vi "Comparation.vi"() -> ()   [LabVIEW 2018]
uses:
  MainFGV/Settings/Advanced/AdvancedConfig.ctl
  Processing/GraphMean/plot_props.ctl
  Processing/GraphMean/axis_props.ctl
  <vilib>/Heliosphere Research LLC/Advanced Plotting Toolkit/api_core/NewPlotScales.ctl
  Processing/results_data.ctl
  Processing/GraphMean/data_mean_plot.ctl
  <vilib>/Analysis/NI_AALPro.lvlib
  <vilib>/Heliosphere Research LLC/Advanced Plotting Toolkit/Advanced Plotting Toolkit.lvlib
panel:
  in  "order":i32=2 caption="Ordem suavização" min=2 max=20
  in  "freq_suav":dbl(slide) caption="Frequência suavização" scale=0.1..0.5
  in  "peakMode":bool
  in  "ranges":T1(array[cluster])=[{"minFreq"=0.0, "maxFreq"=1000.0, "alpha"=20.0}] caption="Ranges de procura de picos" {"alpha" min=0.0 max=100.0 format="%#_6f %"; "maxFreq" format="%#_g Hz"; "minFreq" format="%#_g Hz"}
  in  "Ensaios":path=path "C:/Users/l01481/Desktop/nada"
  in  "channel":i32=1 caption="Canal" min=1 max=4
  in  "stop":bool
  in  "log":bool
  in  "alpha":dbl=0.3 caption="Alpha" format="%#_6f"
  in  "maxFreq":dbl=72.0 caption="Frequência máxima" format="%#_g Hz"
  in  "minFreq":dbl=30.0 caption="Frequência mínima" format="%#_g Hz"
  in  "lowPass":dbl=1000.0 caption="Passa baixa" format="%#_g Hz"
  in  "highPass":dbl=1.0 caption="Passa alta" format="%#_g Hz"
  in  "Filtro":T2(ring)=enum."Passa banda"
  in  "cutoff":dbl=-6.0 caption="Cutoff amplitude [dB]" format="%#_g dB"
  in  "delete":bool
  in  "ok":bool
  in  "validate":bool
  in  "tab":T3(tab)
  out "inert":waveform(dbl)[](graph) caption="Inertância"
  out "hammerSpec":waveform(dbl)(graph) caption="Martelo - Espectro"
  out "acelTime":waveform(dbl)[](graph) caption="Acelerômetros - Sinal no tempo"
  out "hammerTime":waveform(dbl)(graph) caption="Martelo - Sinal no tempo"
  out "meanInert":picture
  out "Picos":cluster{"freqs":dbl[], "Array":dbl[]}[](graph) caption="XY Graph"
  out "Frequências":dbl[][](array[numeric])
  out "Picos 2":cluster{"freqs":dbl[], "Array":dbl[]}[](graph) caption="XY Graph"
  # "Análise modal\n\nAquisição\n\nLink do repositório: https://github.com/LeonardoSirino/ModalAnalysis"
  # "Leonardo Sirino\nSistemas Mecânicos \nT + 55 (41) 3361-6152 | C + 55 (41) 99679-007\nleonardo.sirino@lactec.org.br | www.lactec.org.br"
  # "Configurações para\napresentação"
  # "Configurações para\nprocessamento"
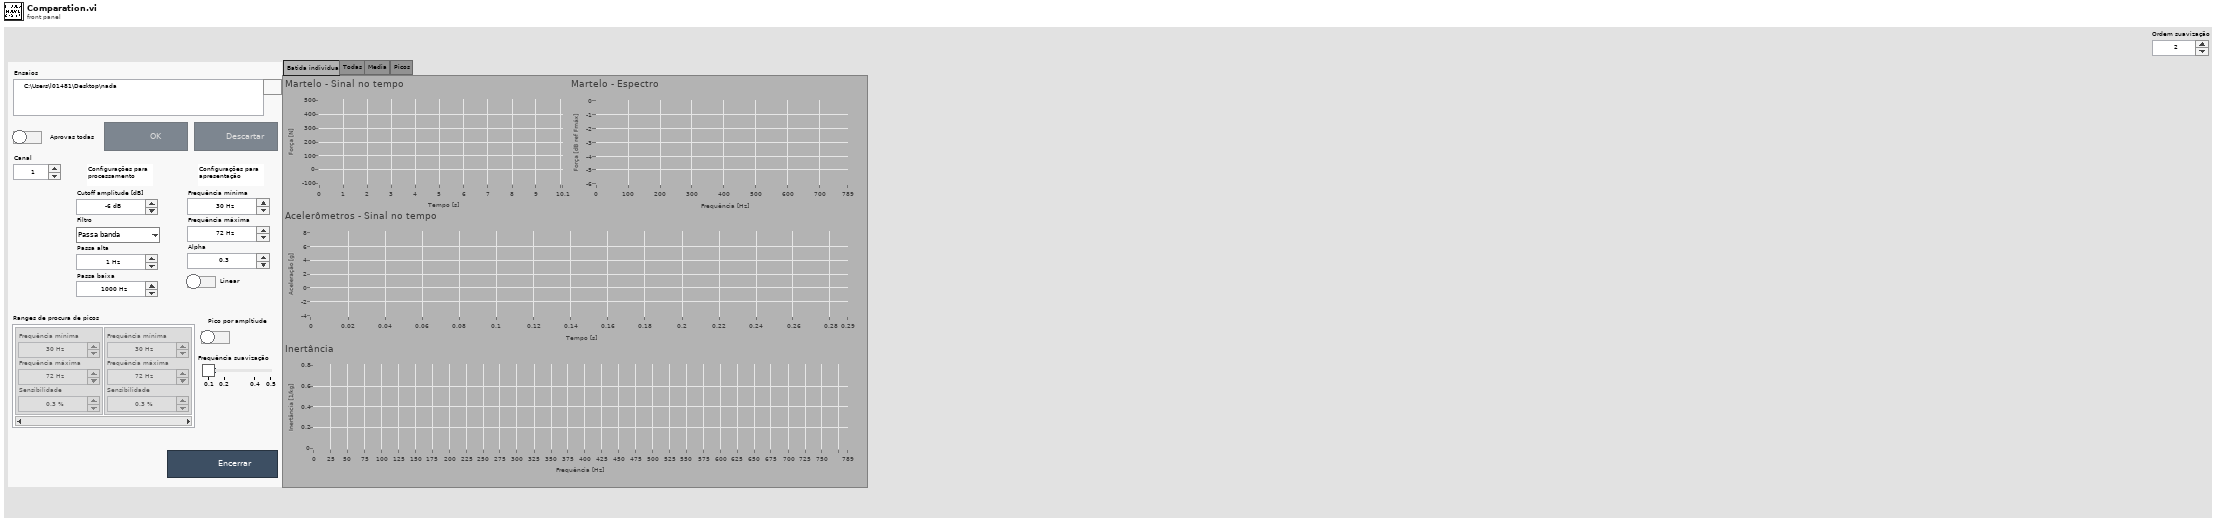
[diagram p1: front panel]
types:
  T1 = cluster{"minFreq":dbl, "maxFreq":dbl, "alpha":dbl}[]
  T2 = enum16{"Desativado", "Passa banda", "Passa alta", "Passa baixa"}
  T3 = enum32{"Batida individual", "Todas", "Media", "Picos"}
  T4 = typedef "plot_props.ctl" = cluster{"x_axis":T5, "y_axis":T5, "y multiplier":dbl, "alpha":dbl, "base_tag":string, "itens_base_name":string, "graph_title":string, "plot_names":string[], "plot_all":bool}
  T5 = typedef "axis_props.ctl" = cluster{"min":dbl, "max":dbl, "label":string, "scale":T6}
  T6 = typedef "Advanced Plotting Toolkit.lvlib/NewPlotScales.ctl" = enum16{"Default", "Linear", "Log", "Symlog"}
  T7 = enum8{"Enabled", "Disabled", "Disabled and Grayed Out"}
  T8 = typedef "AdvancedConfig.ctl" = cluster{"rate":dbl, "duration":dbl, "thr":dbl, "preTrigger":dbl, "cutoff":dbl, "Filtro":enum16{"Desativado", "Passa banda", "Passa alta", "Passa baixa"}, "highPass":dbl, "lowPass":dbl, "updateTime":dbl}
  T9 = typedef "results_data.ctl" = cluster{"config":T8, "hammer":waveform(dbl), "acelerometers":waveform(dbl)[], "hammerIndex":i32}
  T10 = cluster{"seconds since 1Jan1904":timestamp, "data_out":T9}
  T11 = typedef "data_mean_plot.ctl" = cluster{"array":dbl[], "dx":dbl, "x0":dbl}
  T12 = cluster{"seconds since 1Jan1904":timestamp, "data_out":T9}[]
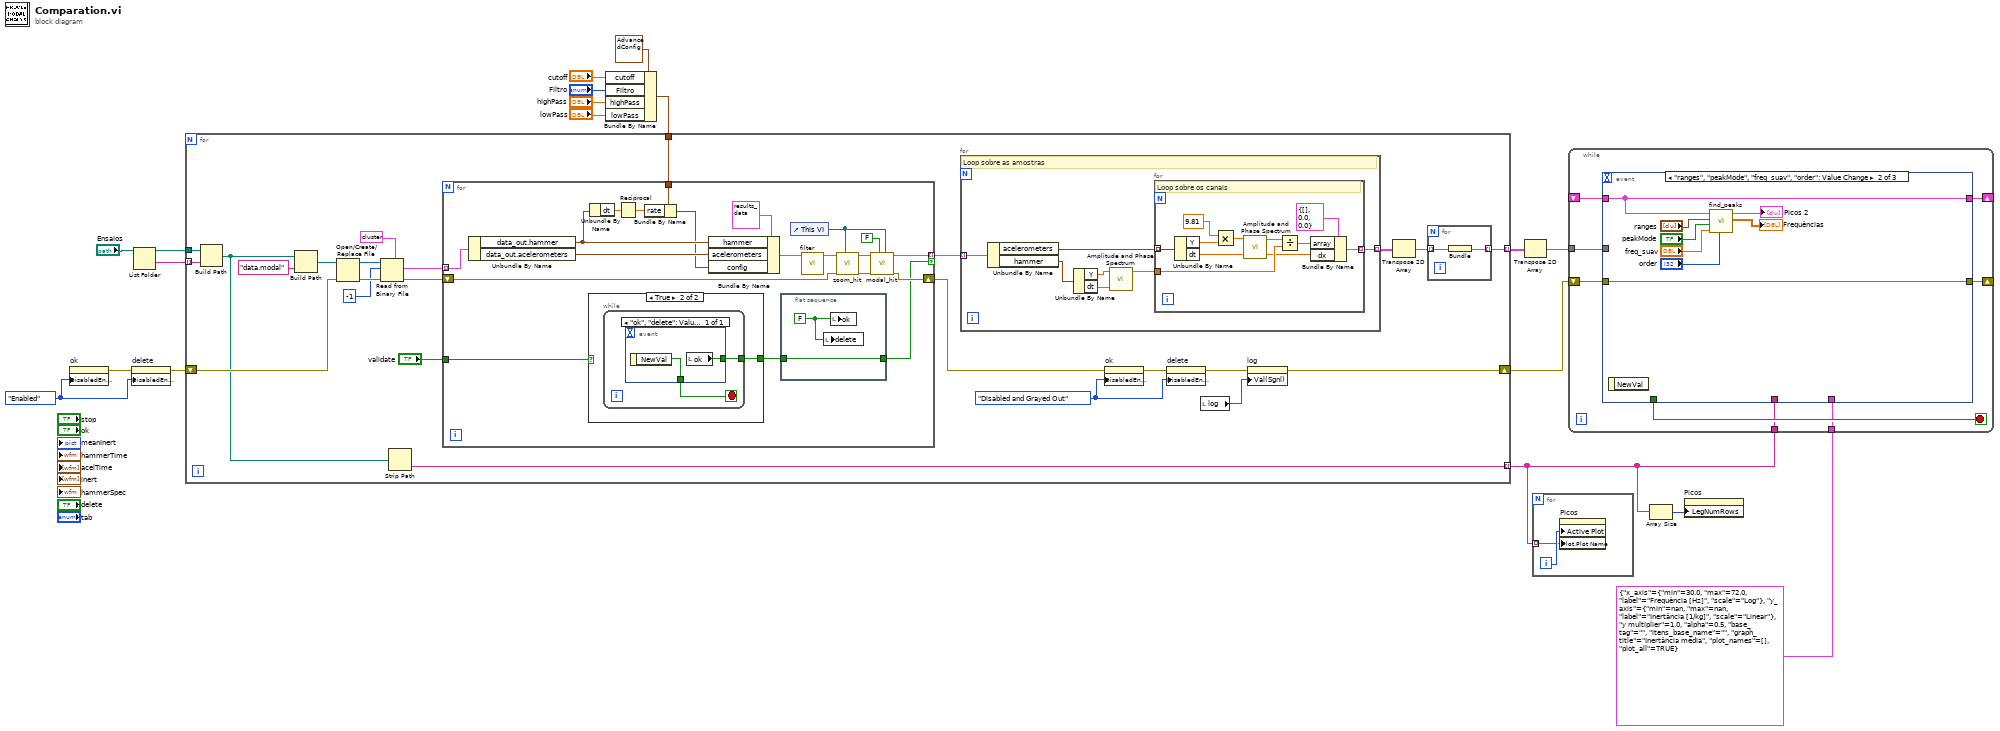
[diagram p0: block diagram]
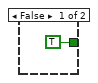
[diagram p2: hidden frame]
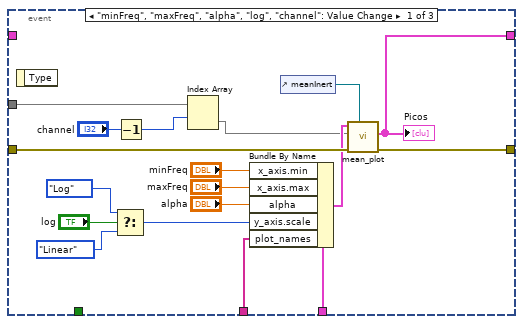
[diagram p3: hidden frame]
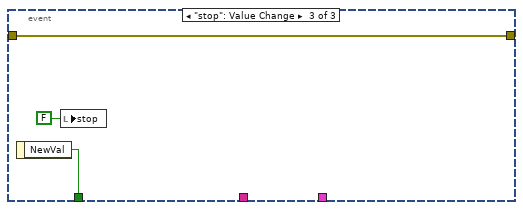
[diagram p4: hidden frame]
diagram:
  w11 = T7."Enabled" ("Disabled")
  n1 = property on="ok" class="Bool (strict)"("DisabledEnum"=w11) -> (error out=w10:errorcluster)  [unwired: 2 in, 1 out]
  n2 = property on="delete" class="Bool (strict)"(error in=w10, "DisabledEnum"=w11) -> (error out=w9:errorcluster)  [unwired: 1 in, 1 out]
  n3 = List Folder(path="Ensaios") -> (path out=w2:path, folder names=w1:string[])  [unwired: 3 in, 2 out]
  n4 = Bundle By Name(cluster=T8 {"rate"=1652.0, "duration"=1.0, "thr"=10.0, "preTrigger"=100.0, "cutoff"=-6.0, "Filtro"=enum."Passa banda", "highPass"=1.0, "lowPass"=1000.0, "updateTime"=50.0} ("config"), "cutoff"="cutoff", "Filtro"="Filtro", "highPass"="highPass", "lowPass"="lowPass") -> (w13:T8)
  n5 = for {
    tunnel: w13 -> [w36]
    tunnel: [w28] -> w8 mode=indexing
    shift-right: [w29] -> w12
    shift-left: w9 -> [w23]
    tunnel: w2 -> [w21]
    tunnel: [w22] -> w6 mode=indexing
    tunnel: w1 -> [w20] mode=indexing
    w25 = T7."Disabled and Grayed Out" ("Disabled")
    n6 = Build Path(base path=w21, name or relative path=w20) -> (appended path=w19:path)
    n7 = Build Path(base path=w19, name or relative path="data.modal") -> (appended path=w42:path)
    n8 = Open/Create/Replace File(file path (use dialog)=w42, error in=w23) -> (refnum out=w41:refnum<file>, error out=w39:errorcluster)  [unwired: 4 in, 1 out]
    n9 = Read from Binary File(5:T10 {"seconds since 1Jan1904"=timestamp(0 s since 1904-01-01), "data_out"={"config"={"rate"=0.0, "duration"=0.0, "thr"=0.0, "preTrigger"=0.0, "cutoff"=0.0, "Filtro"=enum."Desativado", "highPass"=0.0, "lowPass"=0.0, "updateTime"=0.0}, "hammer"={"t0"=timestamp(0 s since 1904-01-01), "dt"=1.0, "Y"=[]}, "acelerometers"=[], "hammerIndex"=0}} ("output cluster"), 8:w39, 10:-1 ("count (1)"), 11:w41) -> (0:w35:errorcluster, 2:w37:T12)  [unwired: 2 in, 2 out]
    n10 = Strip Path(path=w19) -> (name=w22:string)  [unwired: 1 out]
    n11 = for {
      tunnel: w37 -> [w83] mode=indexing
      tunnel: w36 -> [w73]
      shift-right: [w68] -> w27
      shift-left: w35 -> [w69]
      tunnel: [w66] -> w33 mode=indexing if=w65
      tunnel: "validate" -> [w64]
      n12 = Unbundle By Name(w83) -> ("data_out.hammer"=w74:waveform(dbl), "data_out.acelerometers"=w78:waveform(dbl)[])
      n13 = case shown="True" w64 {
        tunnel: [TRUE ("ok") w87] -> w67
        frame False {
        }
        frame True {
          n14 = while {
            tunnel: [w89] -> w87
            stop <- w88 stop-if-true
            n15 = event shown="[0] \"ok\", \"delete\": Value Change" {
              selector: _ -> [_]
              dyn-events: _ -> [_]
              timeout: _ -> [_]
              tunnel: [w90] -> w89
              tunnel: [w91] -> w88
              event "ok", "delete": Value Change {
                n16 = event-data() -> ("NewVal"=w91:bool)  [unwired: 1 in]
                n17 = local read "ok"() -> (w90:bool)
              }
            }
          }
        }
      }
      n18 = Unbundle By Name(w74) -> ("dt"=w72:dbl)
      n19 = Reciprocal(x=w72) -> (1/x=w71:dbl)
      n20 = Bundle By Name(cluster=w73, "rate"=w71) -> (w70:T8)
      n21 = Bundle By Name(cluster=T9 {"config"={"rate"=0.0, "duration"=0.0, "thr"=0.0, "preTrigger"=0.0, "cutoff"=0.0, "Filtro"=enum."Desativado", "highPass"=0.0, "lowPass"=0.0, "updateTime"=0.0}, "hammer"={"t0"=timestamp(0 s since 1904-01-01), "dt"=1.0, "Y"=[]}, "acelerometers"=[], "hammerIndex"=0} ("data_in"), "hammer"=w74, "acelerometers"=w78, "config"=w70) -> (w77:T9)
      n22 = flat-sequence {
        tunnel: w67 -> [w85]
        tunnel: [w85] -> w65
        frame #0 {
          w84 = FALSE ("ok")
          n23 = local write "delete"(w84) -> ()
          n24 = local write "ok"(w84) -> ()
        }
      }
      n25 = control-ref of="This VI"() -> (w76:refnum<vi>)
      n26 = call "filter.vi"("data_in"=w77) -> ("data_out"=w80:T9)  [unwired: 9 in, 1 out]
      n27 = call "zoom_hit.vi"("refVI"=w76, "error in"=w69, "data_in"=w80) -> ("error out"=w81:errorcluster, "data_out"=w82:T9)  [unwired: 7 in]
      n28 = call "modal_hit.vi"("refVI"=w76, "acquisition"=FALSE, "error in"=w81, "data_in"=w82) -> ("error out"=w68:errorcluster, "data_out"=w66:T9)  [unwired: 6 in]
    }
    n29 = for {
      tunnel: w33 -> [w52] mode=indexing
      tunnel: [w46] -> w32 mode=indexing
      # "Loop sobre as amostras"
      n30 = Unbundle By Name(w52) -> ("acelerometers"=w51:waveform(dbl)[], "hammer"=w48:waveform(dbl))
      n31 = Unbundle By Name(w48) -> ("Y"=w49:dbl[], "dt"=w50:dbl)
      n32 = call <vilib>:"Amplitude and Phase Spectrum.vi"("dt"=w50, "Signal (V)"=w49) -> ("Amp Spectrum Mag (Vrms)"=w47:dbl[])  [unwired: 1 in, 2 out]
      n33 = for {
        tunnel: w51 -> [w63] mode=indexing
        tunnel: w47 -> [w57]
        tunnel: [w53] -> w46 mode=indexing
        # "Loop sobre os canais"
        n34 = Unbundle By Name(w63) -> ("Y"=w62:dbl[], "dt"=w59:dbl)
        n35 = Multiply(x=9.81, y=w62) -> (x*y=w60:dbl[])
        n36 = call <vilib>:"Amplitude and Phase Spectrum.vi"("dt"=w59, "Signal (V)"=w60) -> ("df"=w54:dbl, "Amp Spectrum Mag (Vrms)"=w58:dbl[])  [unwired: 1 in, 1 out]
        n37 = Divide(x=w58, y=w57) -> (x/y=w55:dbl[])
        n38 = Bundle By Name(cluster=T11 {"array"=[], "dx"=0.0, "x0"=0.0} ("data_mean_plot"), "array"=w55, "dx"=w54) -> (w53:T11)
      }
    }
    n39 = property on="ok" class="Bool (strict)"(error in=w27, "DisabledEnum"=w25) -> (error out=w26:errorcluster)  [unwired: 1 in, 1 out]
    n40 = property on="delete" class="Bool (strict)"(error in=w26, "DisabledEnum"=w25) -> (error out=w24:errorcluster)  [unwired: 1 in, 1 out]
    n41 = local read "log"() -> (w30:bool)
    n42 = property on="log" class="Bool (strict)"(error in=w24, "Val(Sgnl)"=w30) -> (error out=w29:errorcluster)  [unwired: 1 in, 1 out]
    n43 = Transpose 2D Array(2D array=w32) -> (transposed array=w31:T11[][])
    n44 = for {
      tunnel: w31 -> [w45] mode=indexing
      tunnel: [w44] -> w28 mode=indexing
      n45 = Bundle(w45) -> (w44:cluster{T11[]})  [unwired: 1 in]
    }
  }
  n46 = Transpose 2D Array(2D array=w8) -> (transposed array=w7:cluster{T11[]}[][])
  n47 = for {
    tunnel: w6 -> [w92] mode=indexing
    i -> [w93]
    n48 = property on="Picos" class="XYGraph (strict)"("Active Plot"=w93, "Plot.Plot Name"=w92) -> ()  [unwired: 2 in, 2 out]
  }
  n49 = while {
    shift-right: [w100] -> _
    shift-left: _ -> [w101]
    shift-right: [w99] -> _
    shift-left: w12 -> [w98]
    tunnel: w7 -> [w96]
    tunnel: w6 -> [w95]
    tunnel: T4 {"x_axis"={"min"=30.0, "max"=72.0, "label"="Frequência [Hz]", "scale"=enum."Log"}, "y_axis"={"min"=nan, "max"=nan, "label"="Inertância [1/kg]", "scale"=enum."Linear"}, "y multiplier"=1.0, "alpha"=0.5, "base_tag"="", "itens_base_name"="", "graph_title"="Inertância média", "plot_names"=[], "plot_all"=TRUE} ("plot_properties") -> [w94]
    stop <- w97 stop-if-true
    n50 = event shown="[1] \"ranges\", \"peakMode\", \"freq_suav\", \"order\": Value Change" {
      selector: _ -> [_ _ _]
      dyn-events: _ -> [_ _ _]
      timeout: _ -> [_ _ _]
      tunnel: w101 -> [_ w126 _]
      tunnel: [w105 w126 _] -> w100
      tunnel: [w109 w125 w129] -> w99
      tunnel: w98 -> [w118 w125 w129]
      tunnel: [_ _ w130] -> w97
      tunnel: w96 -> [w108 _ _]
      tunnel: w95 -> [w104 _ _]
      tunnel: w94 -> [w102 _ _]
      event "minFreq", "maxFreq", "alpha", "log", "channel": Value Change {
        n51 = event-data() -> ()  [unwired: 1 in, 1 out]
        n52 = Select(t=NewPlotScales."Log" ("y_axis.scale"), s="log", f=NewPlotScales."Linear" ("y_axis.scale")) -> (s? t:f=w117:T6)
        n53 = Decrement(x="channel") -> (x-1=w103:i32)
        n54 = Index Array(array=w108, index (row)=w103) -> (element=w107:cluster{T11[]}[])  [unwired: 1 in]
        n55 = Bundle By Name(cluster=w102, "x_axis.min"="minFreq", "x_axis.max"="maxFreq", "alpha"="alpha", "y_axis.scale"=w117, "plot_names"=w104) -> (w110:T4)
        n56 = control-ref of="meanInert"() -> (w119:refnum<vi>)
        n57 = call "mean_plot.vi"("ref_picture"=w119, "error in"=w118, "channels"=w107, "plot_properties"=w110) -> ("error out"=w109:errorcluster, "mean_curves"=w105:cluster{"freqs":dbl[], "Array":dbl[]}[])  [unwired: 5 in, 1 out]
        "Picos" <- w105
      }
      event "ranges", "peakMode", "freq_suav", "order": Value Change {
        n58 = event-data() -> ()  [unwired: 1 in, 1 out]
        n59 = call "find_peaks.vi"("order"="order", "freq"="freq_suav", "derivativePeak"="peakMode", "ranges"="ranges", "data"=w126) -> ("freqs"=→"Frequências":dbl[][], "plots"=→"Picos 2":cluster{"Array":dbl[], "Array":dbl[]}[])  [unwired: 3 in, 2 out]
      }
      event "stop": Value Change {
        n60 = event-data() -> ("NewVal"=w130:bool)  [unwired: 1 in]
        n61 = local write "stop"(FALSE ("stop")) -> ()
      }
    }
  }
  n62 = Array Size(array=w6) -> (size(s)=w5:i32)
  n63 = property on="Picos" class="XYGraph (strict)"("LegNumRows"=w5) -> ()  [unwired: 2 in, 2 out]
